vi "Test.vi"   [LabVIEW 2017]
doc: "This VI is called when test mode begins, and will automatically be terminated when it ends. You can add manual or automatic tests and invoke them from the dashboard."
uses:
  <vilib>/Rock Robotics/WPI/DriverStation/WPI_DriverStationRobotMode2.ctl
types:
  T1 = typedef "WPI_DriverStationRobotMode2.ctl" = enum16{"Autonomous Disabled", "Autonomous Enabled", "Teleop Disabled", "Teleop Enabled", "Disconnected", "Finish", "Test Disabled", "Test Enabled", "Emergency Stopped"}
  T2 = typedef "def HARDWARE CTRL info.ctl" = cluster{"DRIVE MOTORS":T3[], "Controller":T6[], "ENCODERS":T8[], "GYRO HARDWARE":T11, "AIR":cluster{"PRESSURE":T14[], "COMPRESSOR":T16, "SOLENOIDS":T17[]}, "MOTORS":T3[], "SERVOS":T20[], "SONAR":T21[], "RELAY":T24[], "LIMIT":T28[]}
  T3 = typedef "def MOTOR info.ctl" = cluster{"Descr":string, "Motor Controller":T4, "PWM ch":T5, "Invert?":bool, "Installed?":bool, "RefName":string, "stack name":string, "remove deadband":bool}
  T4 = typedef "ctrl MOTOR CTRLR SELECT.ctl" = u16
  T5 = typedef "FPGA_DIOPWMChannel.ctl" = enum8{"PWM 0", "PWM 1", "PWM 2", "PWM 3", "PWM 4", "PWM 5", "PWM 6", "PWM 7", "PWM 8", "PWM 9", "PWM MXP 0", "PWM MXP 1", "PWM MXP 2", "PWM MXP 3", "PWM MXP 4", "PWM MXP 5", "PWM MXP 6", "PWM MXP 7", "PWM MXP 8", "PWM MXP 9", "Invalid"}
  T6 = typedef "def USER CONTROL info.ctl" = cluster{"Descr":string, "Installed?":bool, "RefName":string, "JoystickDevice":T7, "Invert Y axis":bool, "Scale":dbl, "AXIS":string, "BUTTONS":string, "POV":string}
  T7 = typedef "WPI_JoystickDeviceEnum.ctl" = enum16{"USB 0", "USB 1", "USB 2", "USB 3", "USB 4", "USB 5"}
  T8 = typedef "def ENCODER info.ctl" = cluster{"Descr":string, "Installed?":bool, "A Channel":T9, "B Channel":T9, "Invert Direction":bool, "Enum":T10, "Gear ratio":dbl, "Cycles per Rev":dbl, "Diameter (in)":dbl[unit], "RefName":string, "stack name":string, "min rate (hz)":dbl, "Samples":u8, "STACK subnames":cluster{"RESET name":string, "STOPPED name":string, "DIRECTION name":string, "RATE name":string, "INSTALLED name":string}}
  T9 = typedef "FPGA_DIOChannel.ctl" = enum8{"DIO 0", "DIO 1", "DIO 2", "DIO 3", "DIO 4", "DIO 5", "DIO 6", "DIO 7", "DIO 8", "DIO 9", "DIO MXP 0", "DIO MXP 1", "DIO MXP 2", "DIO MXP 3", "DIO MXP 4", "DIO MXP 5", "DIO MXP 6", "DIO MXP 7", "DIO MXP 8", "DIO MXP 9", "DIO MXP 10", "DIO MXP 11", "DIO MXP 12", "DIO MXP 13", "DIO MXP 14", "DIO MXP 15", "SPI Port CS1", "SPI Port CS2", "SPI Port CS3", "SPI Port MISO", "SPI Port MOSI", "Invalid"}
  T10 = typedef "WPI_EncoderType.ctl" = enum16{"1x", "2x", "4x"}
  T11 = typedef "def GYRO info.ctl" = cluster{"Descr":string, "Installed?":bool, "SPI Bus":T12, "AnalogChannel":T13, "Calibrate On Open":bool, "Calibrated Center Voltage":dbl, "Calibration Time (s)":dbl, "Sample Rate (Hz)":dbl, "RefName":string, "stack name":string}
  T12 = typedef "spi_bus.ctl" = enum16{"SPI On-Board, CS0", "SPI On-Board, CS1", "SPI On-Board, CS2", "SPI On-Board, CS3", "SPI MXP", "Invalid"}
  T13 = typedef "ctrl ANALOG CHANNEL SELECT.ctl" = enum8{"AI 0", "AI 1", "Invalid"}
  T14 = typedef "def AIR PRESSURE info.ctl" = cluster{"Descr":string, "Installed?":bool, "Channel":T15, "RefName":string, "stack name":string, "MULTIPLIER":dbl, "OFFSET":dbl, "nominal value":dbl, "warning LOW":dbl, "warning HIGH":dbl}
  T15 = typedef "FPGA_AIChannel.ctl" = enum8{"AI 0", "AI 1", "AI 2", "AI 3", "AI MXP 0", "AI MXP 1", "AI MXP 2", "AI MXP 3", "Invalid"}
  T16 = typedef "def COMPRESSOR info.ctl" = cluster{"Descr":string, "Installed?":bool, "Pneumatics Control Module":u8, "RefName":string, "stack name":string}
  T17 = typedef "def SOLENOID info.ctl" = cluster{"Descr":string, "Installed?":bool, "Pneumatics Control Module (0)":u8, "DBL":bool, "SolenoidChannel":T18, "SolenoidChannel":T18, "Default SET":T19, "RefName":string, "Value":string}
  T18 = typedef "WPI_SolenoidChannel.ctl" = enum8{"Solenoid 0", "Solenoid 1", "Solenoid 2", "Solenoid 3", "Solenoid 4", "Solenoid 5", "Solenoid 6", "Solenoid 7", "Invalid"}
  T19 = typedef "WPI_SolenoidValue.ctl" = enum16{"Off", "On", "Forward", "Reverse"}
  T20 = typedef "def SERVO info.ctl" = cluster{"Descr":string, "PWM ch":T5, "Installed?":bool, "Angular range":dbl, "RefName":string, "stack name":string}
  T21 = typedef "def SONAR info.ctl" = cluster{"Descr":string, "Installed?":bool, "Device type":T22, "PING Channel":T9, "ECHO Channel":T9, "RefName":string, "stack name":string, "Samples":i32, "Range Units":T23}
  T22 = typedef "ctrl SONAR DEVICE SELECT.ctl" = enum16{"SRF04 Digital", "MB1010 Digital", "MB1010 Analog", "SRF08 Digital"}
  T23 = typedef "WPI_UltrasonicRangeUnits.ctl" = enum16{"inches", "mm"}
  T24 = typedef "def RELAY info.ctl" = cluster{"Descr":string, "Installed?":bool, "RelayChannel":T25, "Relay Direction":T26, "Relay Value":T27, "RefName":string, "Value":string}
  T25 = typedef "FPGA_DIORelayChannel.ctl" = enum8{"Relay 0", "Relay 1", "Relay 2", "Relay 3", "Invalid"}
  T26 = typedef "WPI_RelayDirection.ctl" = enum16{"Both directions", "Forward only", "Reverse only"}
  T27 = typedef "WPI_RelayValue.ctl" = enum16{"Off", "On", "Forward", "Reverse"}
  T28 = typedef "def LIMIT SWITCH info.ctl" = cluster{"Descr":string, "Installed?":bool, "A Channel":T9, "Normally Closed?":bool, "RefName":string, "stack name":string}
  T29 = typedef "WPI_MotorControlDeviceRef.ctl" = cluster{"DeviceStatus":errorcluster, "Type":T30, "PWM":cluster{"PWM Channel":T5, "DeadBand":T31}, "CAN":cluster{"Device Number":u8, "SetOutput VI Ref":variant, "GetOutput VI Ref":variant, "Enable VI Ref":variant, "Disable VI Ref":variant, "Data":variant}, "Invert":bool, "DIO PWM":cluster{"PWM \"Enable\" Channel":T5, "DIO Channel":T9, "PWM Rate":dbl}}
  T30 = typedef "WPI_MotorControlType.ctl" = enum16{"PWM", "CAN", "DIO PWM"}
  T31 = typedef "WPI_PWMDeadband.ctl" = cluster{"Name":string, "maxPositivePwm":i32, "minPositivePwm":i32, "centerPwm":i32, "maxNegativePwm":i32, "minNegativePwm":i32, "angularRange":u16}
  T32 = typedef "WPI_ServoDeviceRef.ctl" = cluster{"DeviceStatus":errorcluster, "PWM Channel":T5, "DeadBand":T31}
  T33 = typedef "WPI_RelayDevRef.ctl" = cluster{"DevStatus":errorcluster, "Relay Channel":T25, "Relay Direction":T26}
  T34 = typedef "WPI_JoystickDevRef.ctl" = cluster{"Device":T7}
  T35 = typedef "WPI_EncoderDevRef.ctl" = cluster{"DevStatus":errorcluster, "EncoderIndex":T36, "CounterIndex":T37, "DistancePerCount":dbl, "Decoding Type":T10}
  T36 = typedef "FPGA_EncoderIdx.ctl" = enum8{"Enc 0", "Enc 1", "Enc 2", "Enc 3", "Enc 4", "Enc 5", "Enc 6", "Enc 7", "Invalid"}
  T37 = typedef "FPGA_CounterCtrSystemIndex.ctl" = enum8{"Ctr 0", "Ctr 1", "Ctr 2", "Ctr 3", "Ctr 4", "Ctr 5", "Ctr 6", "Ctr 7", "Invalid"}
  T38 = typedef "WPI_UltrasonicDeviceRef.ctl" = cluster{"DevStatus":errorcluster, "Ping Channel":T9, "Echo Channel":T9, "CntIndex":T37}
  T39 = typedef "WPI_SwitchDevRef.ctl" = cluster{"DevStatus":errorcluster, "DIO Channel":T9, "CntIndex":T37, "Normally Closed":bool}
  T40 = typedef "WPI_AnalogChannelDevRef.ctl" = cluster{"DevStatus":errorcluster, "Analog Channel":T15}
  T41 = typedef "WPI_RobotDriveDevRef.ctl" = cluster{"DevStatus":errorcluster, "Motors[]":T29[], "Square Inputs":bool, "Max Output":dbl}
  T42 = cluster{"JoystickDevRef":T34, "RobotDriveDevRef":T41}
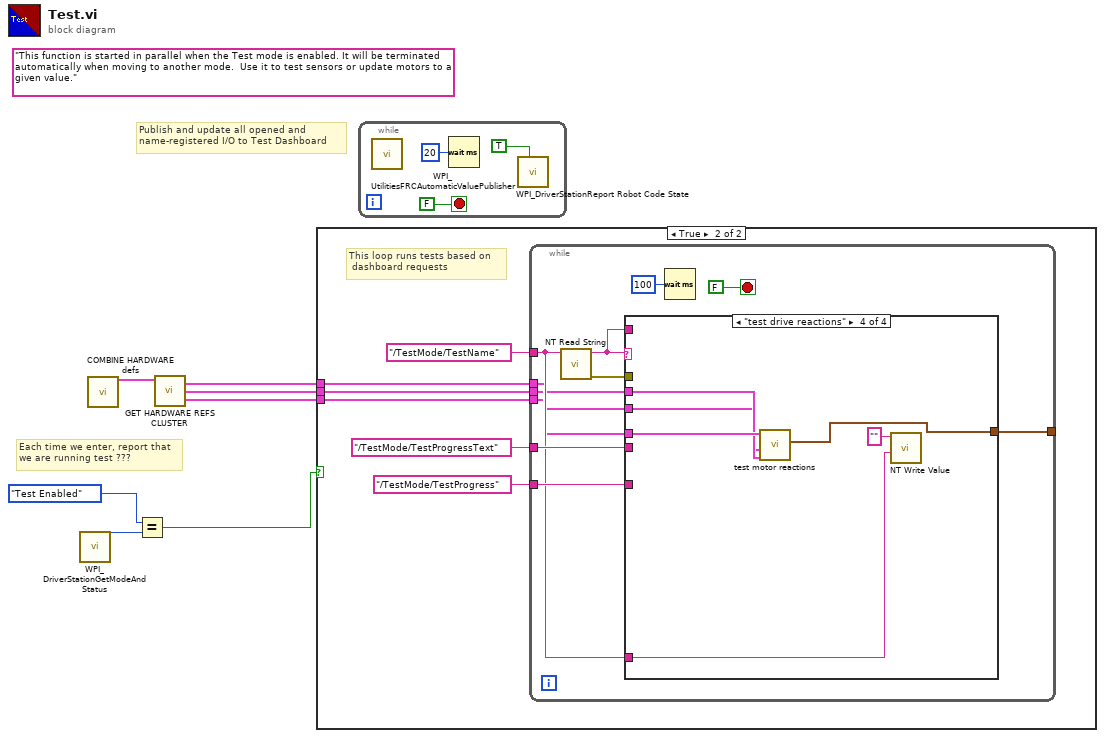
[diagram p0: block diagram]
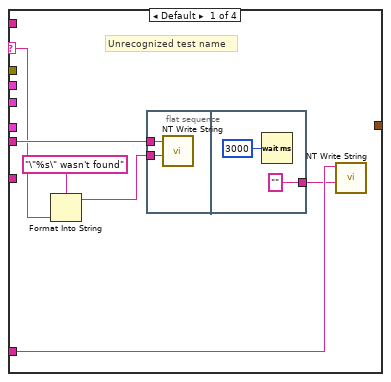
[diagram p3: hidden frame]
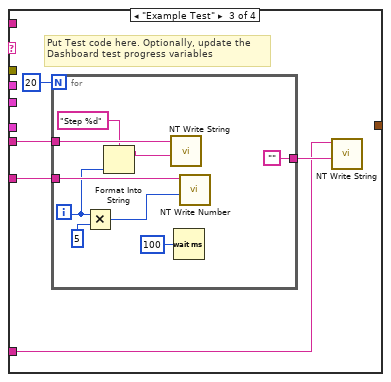
[diagram p5: hidden frame]
diagram:
  (unwired) "This function is started in parallel when the Test mode is enabled. It will be terminated automatically when moving to another mode.  Use it to test sensors or update motors to a given value."
  # "Publish and update all opened and\nname-registered I/O to Test Dashboard"
  # "Each time we enter, report that\nwe are running test ???"
  n1 = call <vilib>:"WPI_DriverStationGetModeAndStatus.vi"() -> ("Robot Mode"=w3:T1)  [unwired: 10 in, 1 out]
  n2 = call "COMBINE HARDWARE defs.vi"() -> ("HARDWARE out"=w7:T2)  [unwired: 10 in, 1 out]
  n3 = Equal?(x=WPI_DriverStationRobotMode2."Test Enabled" ("Robot Mode"), y=w3) -> (x = y?=w1:bool)
  n4 = call "GET HARDWARE REFS CLUSTER.vi"("HARDWARE cluster"=w7) -> ("REF OUTPUT"=w4:cluster{T29[], T32[], T33[]}, "REF INPUT"=w5:cluster{T34[], T35[], T38[], T39[], T40[]}, "REF DRIVE JOYSTICK"=w6:T42)  [unwired: 8 in]
  n5 = case shown="True" w1 {
    tunnel: w6 -> [_ w10]
    tunnel: w5 -> [_ w9]
    tunnel: w4 -> [_ w8]
    frame False {
    }
    frame True {
      # "This loop runs tests based on \n dashboard requests"
      n6 = while {
        tunnel: "/TestMode/TestName" ("Name") -> [w19]
        tunnel: "/TestMode/TestProgressText" ("Name") -> [w22]
        tunnel: "/TestMode/TestProgress" ("Name") -> [w21]
        tunnel: w10 -> [w17]
        tunnel: w9 -> [w16]
        tunnel: w8 -> [w15]
        tunnel: [w14] -> _
        stop <- FALSE stop-if-true
        n7 = call <vilib>:"NT Read String.vi"("Name"=w19) -> ("error out"=w18:errorcluster, "String"=w20:string)  [unwired: 9 in]
        n8 = case shown="\"test drive reactions\"" w20 {
          selector: w20 -> [w29 _ _ _]
          tunnel: w19 -> [w26 _ w35 w51]
          tunnel: w22 -> [w30 _ w38 _]
          tunnel: w21 -> [_ _ w39 _]
          tunnel: w20 -> [_ _ _ _]
          tunnel: w18 -> [_ _ _ _]
          tunnel: w17 -> [_ _ _ w54]
          tunnel: w16 -> [_ _ _ w53]
          tunnel: w15 -> [_ _ _ w52]
          tunnel: [_ _ _ w49] -> w14
          frame Default {
            # "Unrecognized test name"
            n9 = Format Into String(format string="\"%s\" wasn't found" ("Name"), w29) -> (resulting string=w28:string)  [unwired: 2 in, 1 out]
            n10 = flat-sequence {
              tunnel: w30 -> [w31]
              tunnel: w28 -> [w32]
              tunnel: ["" ("Name")] -> w25
              frame #0 {
                n11 = call <vilib>:"NT Write String.vi"("String"=w32, "Name"=w31) -> ()  [unwired: 9 in, 1 out]
              }
              frame #1 {
                n12 = Wait (ms)(milliseconds to wait=u32 3000) -> ()  [unwired: 1 out]
              }
            }
            n13 = call <vilib>:"NT Write String.vi"("String"=w25, "Name"=w26) -> ()  [unwired: 9 in, 1 out]
          }
          frame "" {
            # "No test to run"
          }
          frame "Example Test" {
            # "Put Test code here. Optionally, update the\nDashboard test progress variables"
            n14 = for {
              N: 20 -> [_]
              tunnel: w39 -> [w48]
              tunnel: w38 -> [w46]
              tunnel: ["" ("String")] -> w36
              i -> [w43]
              n15 = Multiply(x=w43, y=u32 5 ("milliseconds to wait")) -> (x*y=w44:u32)
              n16 = Format Into String(format string="Step %d", w43) -> (resulting string=w41:string)  [unwired: 2 in, 1 out]
              n17 = call <vilib>:"NT Write String.vi"("String"=w41, "Name"=w46) -> ()  [unwired: 9 in, 1 out]
              n18 = Wait (ms)(milliseconds to wait=u32 100) -> ()  [unwired: 1 out]
              n19 = call <vilib>:"NT Write Number.vi"("Numeric"=w44, "Name"=w48) -> ()  [unwired: 9 in, 1 out]
            }
            n20 = call <vilib>:"NT Write String.vi"("String"=w36, "Name"=w35) -> ()  [unwired: 9 in, 1 out]
          }
          frame "test drive reactions" {
            n21 = call "test motor reactions.vi"("REF INPUT"=w53, "REF OUTPUT"=w52, "REF DRIVE JOYSTICK"=w54) -> ("Cluster"=w49:cluster{"LEFT":dbl, "RIGHT":dbl})  [unwired: 8 in]
            n22 = call-poly <vilib>:"NT Write Value.vi"("String"=w51, "Name"="") -> ()  [unwired: 9 in, 1 out]
          }
        }
        n23 = Wait (ms)(milliseconds to wait=u32 100) -> ()  [unwired: 1 out]
      }
    }
  }
  n24 = while {
    stop <- FALSE stop-if-true
    n25 = call <vilib>:"WPI_UtilitiesFRCAutomaticValuePublisher.vi"() -> ()  [unwired: 12 in]
    n26 = Wait (ms)(milliseconds to wait=u32 20) -> ()  [unwired: 1 out]
    n27 = call <vilib>:"WPI_DriverStationReport Robot Code State.vi"("Test"=TRUE ("Autonomous")) -> ()  [unwired: 10 in, 1 out]
  }
